vi "SetBaseTime.vi"(8 "error in":errorcluster, 11 "Cycles":T1={"DELICATE"=10.0, "LOW"=10.0, "MEDIUM"=10.0, "HIGH"=10.0} {"HIGH" min=10.0 max=90.0 step=1.0; "MEDIUM" min=10.0 max=90.0 step=1.0; "LOW" min=10.0 max=90.0 step=1.0; "DELICATE" min=10.0 max=90.0 step=1.0}) -> (0 "error out":errorcluster, 3 "TimeData":string)   [LabVIEW 2023]
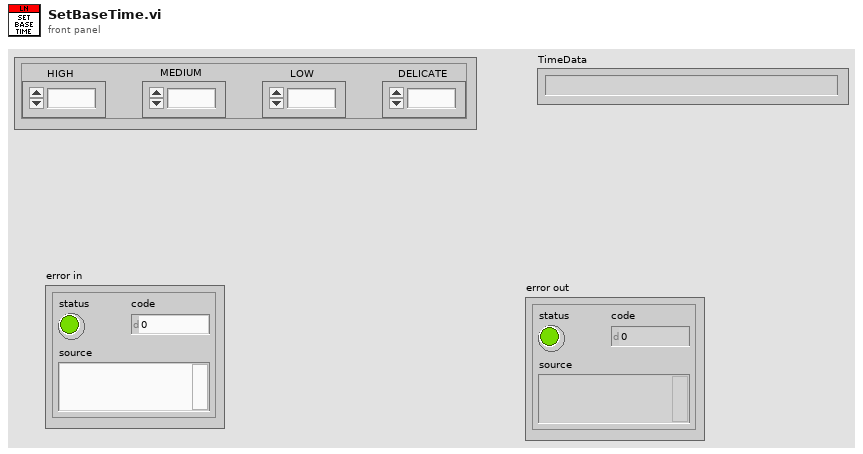
[diagram p1: front panel]
types:
  T1 = cluster{"DELICATE":dbl, "LOW":dbl, "MEDIUM":dbl, "HIGH":dbl}
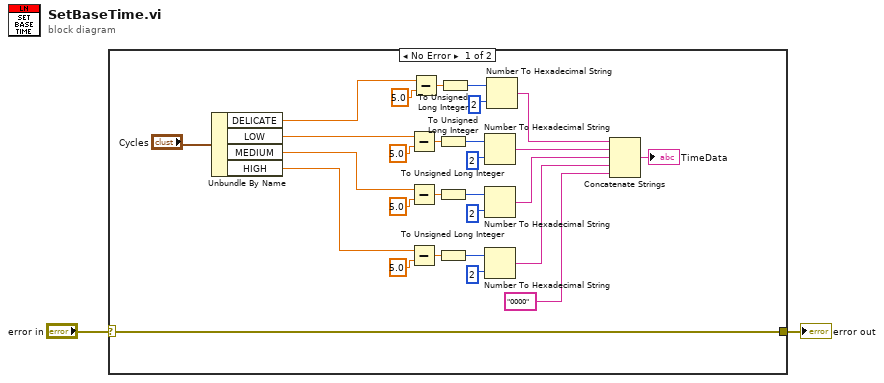
[diagram p0: block diagram]
diagram:
  n1 = case shown="No Error" "error in" {
    selector: "error in" -> [w3 w31]
    tunnel: [w3 w31] -> w1
    frame No Error {
      n2 = Unbundle By Name("Cycles") -> ("DELICATE"=w7:dbl, "LOW"=w6:dbl, "MEDIUM"=w5:dbl, "HIGH"=w4:dbl)
      n3 = Subtract(x=w6, y=5.0) -> (x-y=w25:dbl)
      n4 = Subtract(x=w5, y=5.0) -> (x-y=w20:dbl)
      n5 = Subtract(x=w4, y=5.0) -> (x-y=w17:dbl)
      n6 = Subtract(x=w7, y=5.0) -> (x-y=w28:dbl)
      n7 = To Unsigned Long Integer(number=w25) -> (unsigned 32bit integer=w26:u32)
      n8 = To Unsigned Long Integer(number=w20) -> (unsigned 32bit integer=w19:u32)
      n9 = To Unsigned Long Integer(number=w17) -> (unsigned 32bit integer=w18:u32)
      n10 = To Unsigned Long Integer(number=w28) -> (unsigned 32bit integer=w27:u32)
      n11 = Number To Hexadecimal String(1:i16 2 ("width (-)"), 2:w26) -> (0:w13:string)
      n12 = Number To Hexadecimal String(1:i16 2 ("width (-)"), 2:w19) -> (0:w12:string)
      n13 = Number To Hexadecimal String(1:i16 2 ("width (-)"), 2:w18) -> (0:w11:string)
      n14 = Number To Hexadecimal String(1:i16 2 ("width (-)"), 2:w27) -> (0:w14:string)
      n15 = Concatenate Strings(w14, w13, w12, w11, "0000" ("string")) -> (→"TimeData":string)
    }
    frame Error {
    }
  }
  "error out" <- w1
